vi "get_config_cluster.vi"(8 "error in (no error)":errorcluster, 11 "TrajectoryDL110413StraightLine in":refnum<class "TrajectoryDL110413StraightLine.lvclass">) -> (0 "error out":errorcluster, 2 "config cluster (variant)":variant, 3 "TrajectoryDL110413StraightLine out":refnum<class "TrajectoryDL110413StraightLine.lvclass">)   [LabVIEW 2010, in "TrajectoryDL110413StraightLine.lvclass"]
uses:
  TrajectoryDL110413StraightLine.lvclass
  TrajectoryDL110413StraightLine.lvclass/TrajectoryDL110413StraightLine.ctl
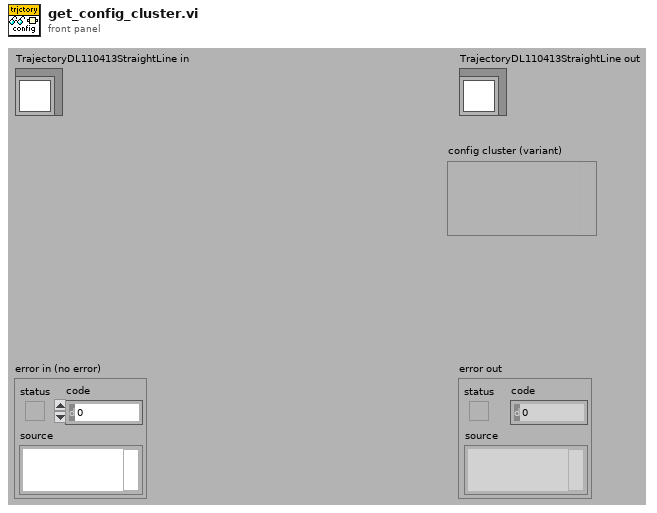
[diagram p1: front panel]
types:
  T1 = typedef "TrajectoryDL110413StraightLine.lvclass/config_data_cluster.ctl" = cluster{"xpaths":cluster{"x offset":string, "y offset":string, "z offset":string}}
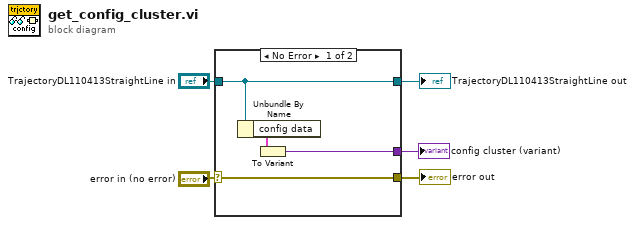
[diagram p0: block diagram]
diagram:
  n1 = case shown="No Error" "error in (no error)" {
    selector: "error in (no error)" -> [w7 w10]
    tunnel: "TrajectoryDL110413StraightLine in" -> [w6 w11]
    tunnel: [w8 _] -> w4
    tunnel: [w7 w10] -> w2
    tunnel: [w6 w11] -> w1
    frame No Error {
      n2 = Unbundle By Name(w6) -> ("config data"=w9:T1)
      n3 = To Variant(anything=w9) -> (Variant=w8:variant)
    }
    frame Error {
    }
  }
  "error out" <- w2
  "TrajectoryDL110413StraightLine out" <- w1
  "config cluster (variant)" <- w4
